vi "Arm.vi"(8 "error in (no error)":errorcluster, 11 "RP Instrument in":refnum<class "RP Instrument.lvclass">) -> (0 "error out":errorcluster, 3 "RP Instrument out":refnum<class "RP Instrument.lvclass">)   [LabVIEW 2024, in "RP Instrument.lvclass"]
uses:
  RP Instrument.lvclass
  RP Instrument.lvclass/RP Instrument.ctl
  RP Command.ctl
  Read Post-trigger samples.vi
  RP Communicator/RP Communicator.lvclass
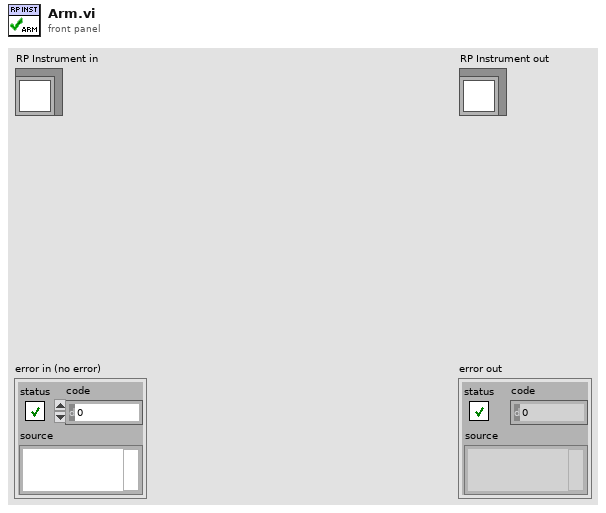
[diagram p1: front panel]
types:
  T1 = typedef "RP Command.ctl" = enum16{"Reset", "Read IDN", "Stop server", "Get status", "Get temperature", "Connect client", "Arm", "Software trigger", "Get whole buffer", "Get chunk", "System call", "Get config", "Set config", "Recieve data", "Recieve Calibartion", "Transmit data"}
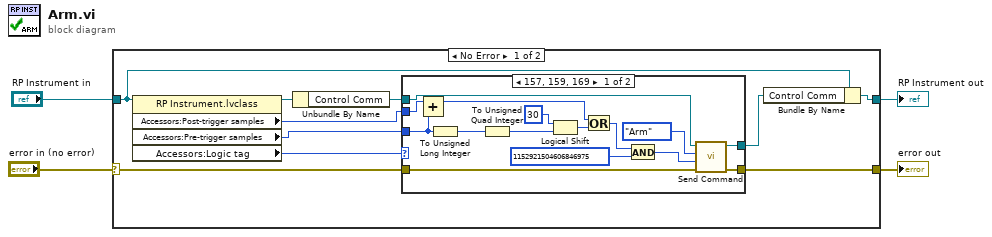
[diagram p0: block diagram]
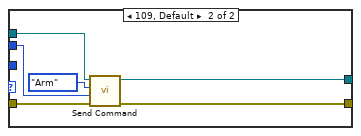
[diagram p2: hidden frame]
diagram:
  n1 = case shown="No Error" "error in (no error)" {
    selector: "error in (no error)" -> [w12 w37]
    tunnel: [w11 w37] -> w3
    tunnel: [w10 w36] -> w1
    tunnel: "RP Instrument in" -> [w14 w36]
    frame No Error {
      n2 = property class="RP Instrument.lvclass"(reference=w14) -> (reference out=w8:refnum<class "RP Instrument.lvclass">, "Accessors:Post-trigger samples"=w6:u64, "Accessors:Pre-trigger samples"=w5:u64, "Accessors:Logic tag"=w7:u16)  [unwired: 1 in, 1 out]
      n3 = Unbundle By Name(w8) -> ("Control Comm"=w13:refnum<class "RP Communicator.lvclass">)
      n4 = case shown="157, 159, 169" w7 {
        tunnel: w13 -> [w29 w35]
        tunnel: w12 -> [w27 w33]
        tunnel: [w26 w32] -> w11
        tunnel: [w25 w31] -> w9
        tunnel: w6 -> [w20 w30]
        tunnel: w5 -> [w15 _]
        frame 157, 159, 169 {
          n5 = Add(x=w20, y=w15) -> (x+y=w16:u64)
          n6 = To Unsigned Long Integer(number=w15) -> (unsigned 32bit integer=w24:u32)
          n7 = To Unsigned Quad Integer(1:w24) -> (0:w22:u64)
          n8 = Logical Shift(y=i16 30, x=w22) -> (x << y=w21:u64)
          n9 = Or(x=w16, y=w21) -> (x .or. y?=w18:u64)
          n10 = And(x=w18, y=u64 1152921504606846975 ("value")) -> (x .and. y?=w17:u64)
          n11 = call-dynamic "Send Command.vi"("error in (no error)"=w27, "Command payload"=w17, "Command number"=RP_Command."Arm", "RP Communicator in"=w29) -> ("error out"=w26:errorcluster, "RP Communicator out"=w25:refnum<class "RP Communicator.lvclass">)  [unwired: 6 in]
        }
        frame 109, Default {
          n12 = call-dynamic "Send Command.vi"("error in (no error)"=w33, "Command payload"=w30, "Command number"=RP_Command."Arm", "RP Communicator in"=w35) -> ("error out"=w32:errorcluster, "RP Communicator out"=w31:refnum<class "RP Communicator.lvclass">)  [unwired: 6 in]
        }
      }
      n13 = Bundle By Name(cluster=w14, "Control Comm"=w9) -> (w10:refnum<class "RP Instrument.lvclass">)
    }
    frame Error {
    }
  }
  "error out" <- w3
  "RP Instrument out" <- w1
